vi "Stop Core.vi"(10 "final error code":i32, 11 "VIStore in":refnum<class "VIStore.lvclass">) -> (3 "VIStore out":refnum<class "VIStore.lvclass">)   [LabVIEW 2015, in "VI App Store.lvlib" / "VIStore.lvclass"]
doc: "(<B>Filename</B>: Actor Framework.lvlib:Actor.lvclass:Stop Core.vi)\n\nDefines what the actor does before it stops. Use the <B>final error code</B> input to determine whether the actor shut down in response to an error.\n\nBy default, this method does nothing. A descendant class may override it to define behavior, such as shutting down any processes the actor initiated in its override of the Actor Core method."
uses:
  VIStore.lvclass
  VIStore.lvclass/VIStore.ctl
  <vilib>/ActorFramework/Actor/Actor.lvclass
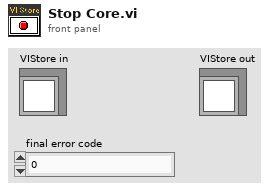
[diagram p1: front panel]
types:
  T1 = typedef "Item Actor.lvlib/Settings.lvclass/Settings Data.ctl" = cluster{"Categories Path":path, "Resizable":bool}
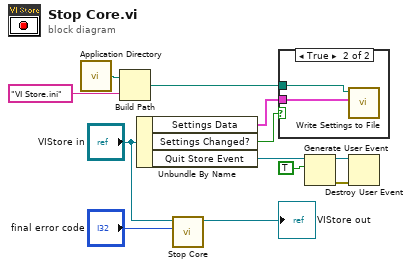
[diagram p0: block diagram]
diagram:
  n1 = call <vilib>:"Application Directory.vi"() -> ("Application Directory"=w5:path)
  n2 = Build Path(base path=w5, name or relative path="VI Store.ini") -> (appended path=w3:path)
  n3 = Unbundle By Name("VIStore in") -> ("Settings Data"=w2:T1, "Settings Changed?"=w1:bool, "Quit Store Event"=w9:refnum<user-event>)
  n4 = call-parent "Stop Core.vi"("final error code"="final error code", "Actor in"="VIStore in") -> ("Actor out"=→"VIStore out":refnum<class "VIStore.lvclass">)  [unwired: 9 in]
  n5 = case shown="True" w1 {
    tunnel: w3 -> [_ w14]
    tunnel: w2 -> [_ w13]
    frame False {
    }
    frame True {
      n6 = call "Write Settings to File.vi"("Settings Data"=w13, "appended path"=w14) -> ()  [unwired: 9 in, 1 out]
    }
  }
  n7 = Generate User Event(user event=w9, event data cluster=TRUE ("event data")) -> (user event out=w6:refnum<user-event>, error out=w7:errorcluster)  [unwired: 2 in]
  n8 = Destroy User Event(user event=w6, error in=w7) -> ()  [unwired: 1 out]
